vi "Extract Data.vi"(8 "Error In":errorcluster, 11 "Folder Path":path) -> (0 "Error Out":errorcluster)   [LabVIEW 2019, in "AnalysisSupport.lvlib"]
uses:
  AnalysisSupport.lvlib
  <vilib>/regexp/Match Regular Expression.xnode
  <vilib>/Analysis/NI_AALBase.lvlib
  CollectionSupport.lvlib
panel:
  out "SPL Values":dbl[](array[numeric])
  out "PTP Values":dbl[](array[numeric])
  out "Pressure Values":dbl[](array[numeric])
  out "MFR Values":dbl[](array[numeric])
  out "File Contents":string[][](array[string])
  out "File Index":i32
  out "File Match":bool
  out "Row Index":i32
  out "SPL Match":bool
  out "PTP Match":bool
  out "Pressure/SGP Match":bool
  out "MFR Match":bool
  out "All Files in Dir":path[](array[path])
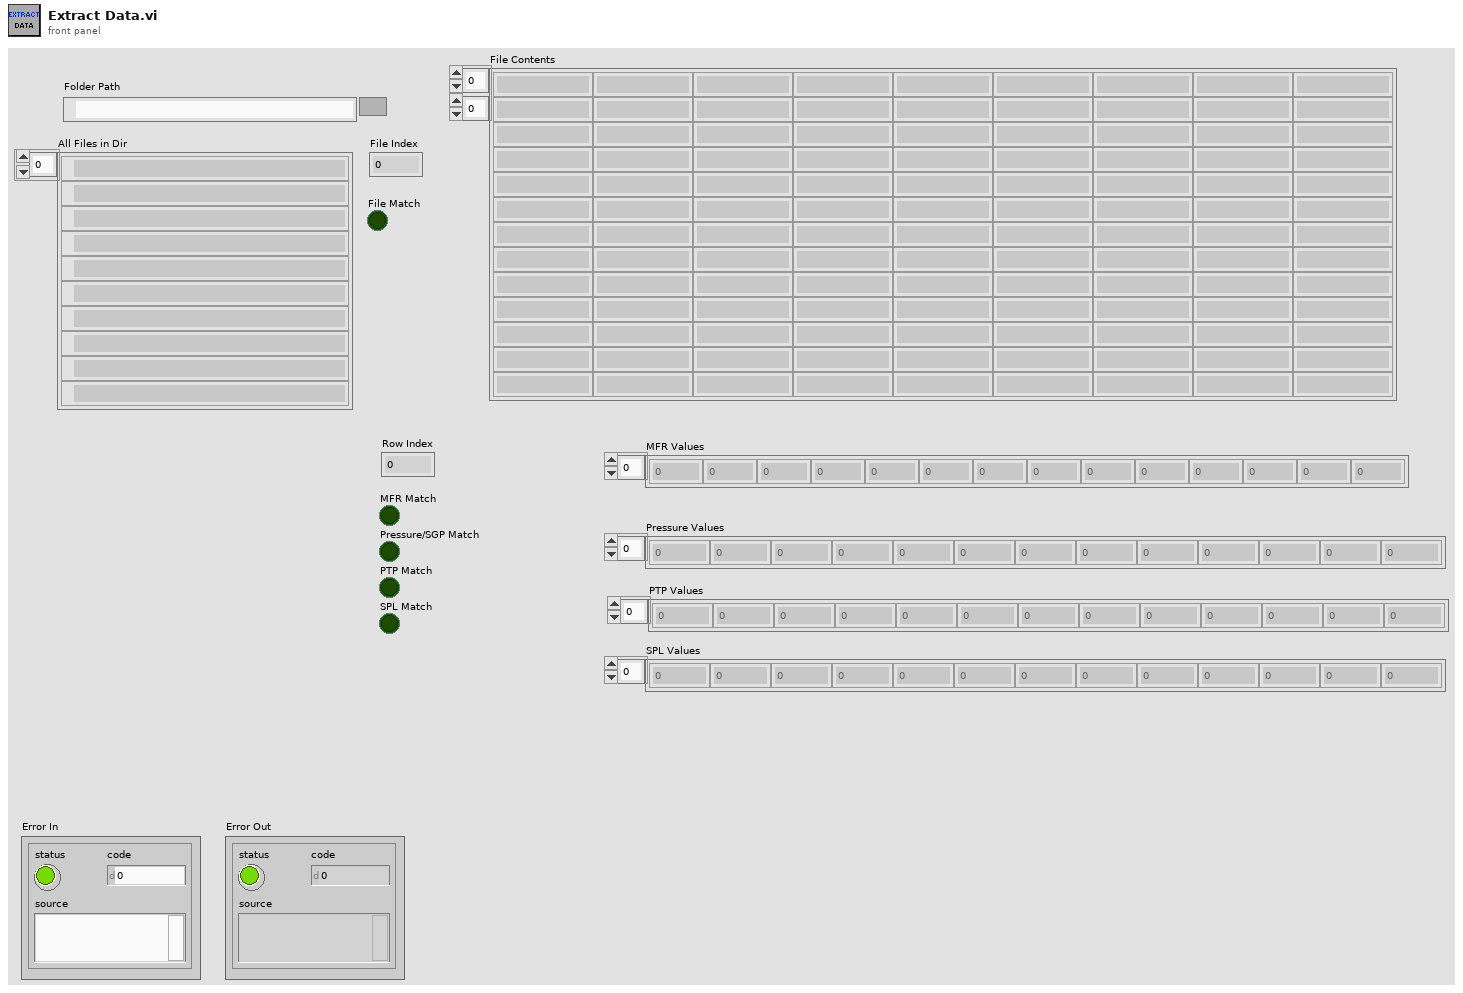
[diagram p1: front panel]
types:
  T1 = enum16{"open", "replace", "create", "open or create", "replace or create", "replace or create with confirmation"}
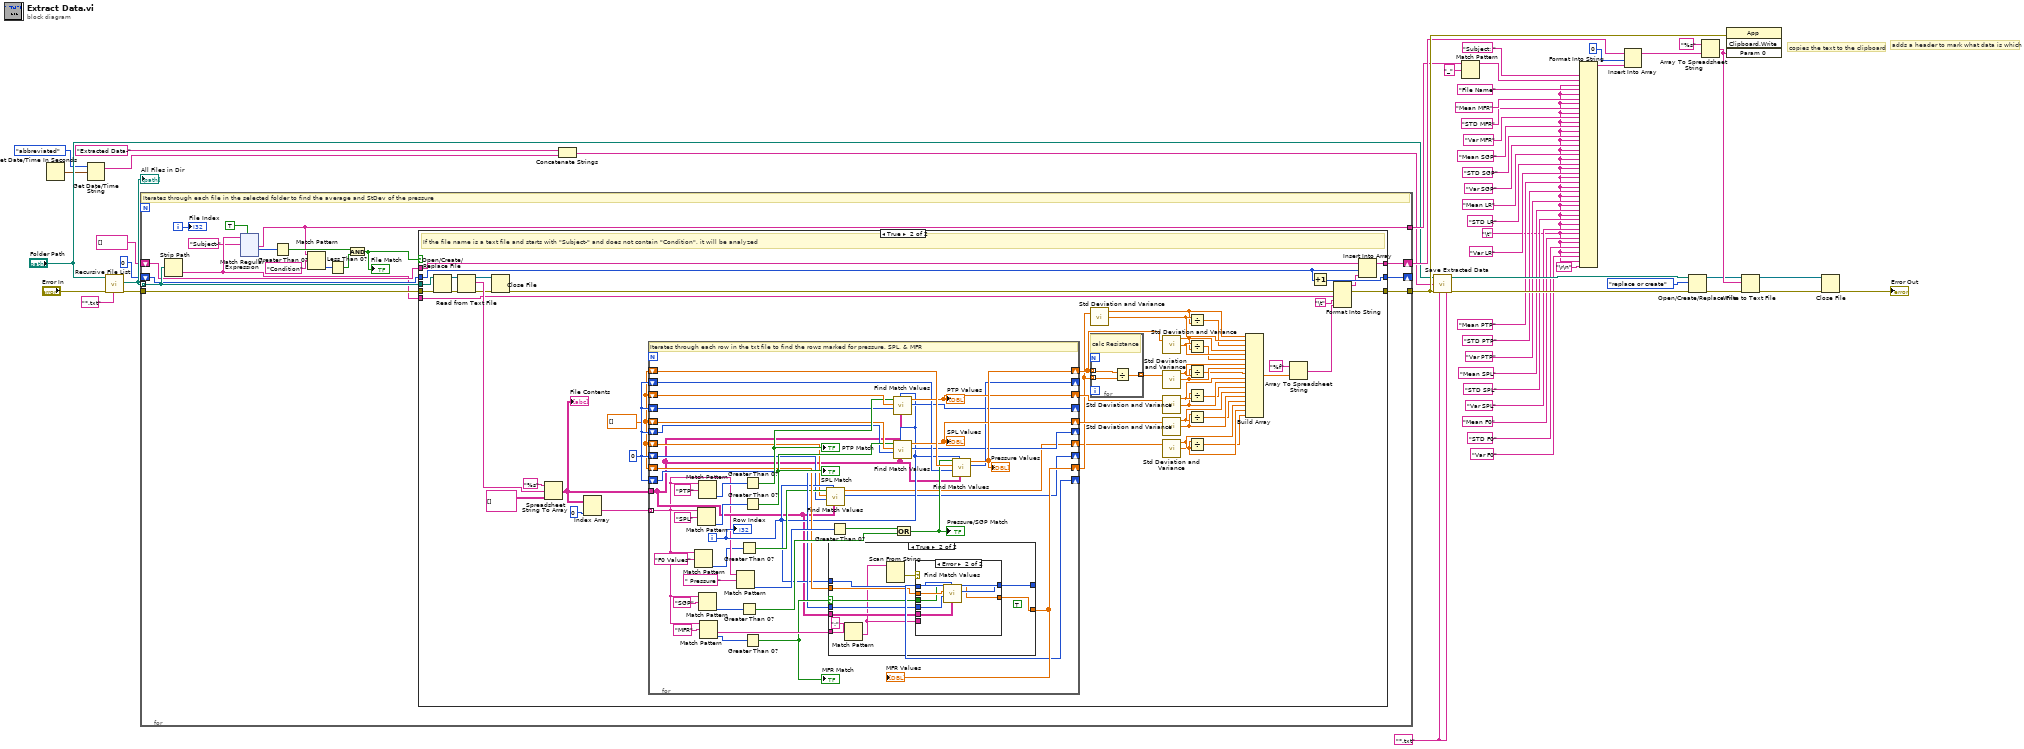
[diagram p0: block diagram]
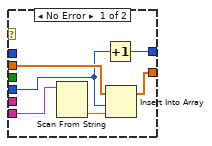
[diagram p4: hidden frame]
diagram:
  w7 = "\t"
  w42 = "*.txt" ("pattern label")
  # "adds a header to mark what data is which"
  # "copies the text to the clipboard"
  n1 = Get Date/Time In Seconds() -> (seconds since 1Jan1904=w5:timestamp)
  n2 = Get Date/Time String(date format (0)=enum16{"short", "long", "abbreviated"}."abbreviated", seconds (now)=w5) -> (date string=w3:string)  [unwired: 1 in, 1 out]
  n3 = call <vilib>:"Recursive File List.vi"("pattern"="*.txt", "error in (no error)"="Error In", "Folder Path"="Folder Path") -> ("error out"=w51:errorcluster, "All Files in Dir"=w52:path[])  [unwired: 4 in, 3 out]
  "All Files in Dir" <- w52
  n4 = for {
    tunnel: w51 -> [w70]
    tunnel: w52 -> [w69] mode=indexing
    shift-right: [w71] -> w38
    shift-left: string[] [] -> [w65]
    shift-right: [w67] -> _
    shift-left: 0 ("index") -> [w68]
    tunnel: [w66] -> w41
    tunnel: [w55] -> w35
    i -> [w54]
    # "Iterates through each file in the selected folder to find the average and StDev of the pressure"
    n5 = Strip Path(path=w69) -> (name=w58:string)  [unwired: 1 out]
    n6 = xnode "Match Regular Expression"("input string"=w58, "regular expression"="Subject-", "ignore case? (F)"=TRUE) -> ("after match"=w55:string, "offset past match"=w56:i32)  [unwired: 3 in, 3 out]
    n7 = Greater Than 0?(x=w56) -> (x > 0?=w62:bool)
    n8 = Match Pattern(string=w55, regular expression="Condition") -> (offset past match=w60:i32)  [unwired: 1 in, 3 out]
    n9 = Less Than 0?(x=w60) -> (x < 0?=w61:bool)
    n10 = And(x=w62, y=w61) -> (x .and. y?=w63:bool)
    "File Match" <- w63
    n11 = case shown="True" w63 {
      tunnel: [w188 w224] -> w71
      tunnel: w70 -> [w186 w227]
      tunnel: w65 -> [w188 w225]
      tunnel: w69 -> [_ w226]
      tunnel: w68 -> [w187 w223]
      tunnel: [w187 w222] -> w67
      tunnel: w58 -> [_ w216]
      tunnel: [w186 w213] -> w66
      frame False {
        # "If a text file doesn't match what we are looking for, nothing happens"
      }
      frame True {
        w191 = 0 ("index")
        w190 = dbl[] [] ("Array")
        # "If the file name is a text file and starts with \"Subject-\" and does not contain \"Condition\", it will be analyzed"
        n12 = Open/Create/Replace File(file path (use dialog)=w226, error in=w227) -> (refnum out=w238:refnum<file>, error out=w237:errorcluster)  [unwired: 4 in, 1 out]
        n13 = Read from Text File(file (use dialog)=w238, error in=w237) -> (refnum out=w236:refnum<file>, text=w235:string, error out=w215:errorcluster)  [unwired: 2 in, 1 out]
        n14 = Close File(refnum=w236, error in=w215) -> (error out=w214:errorcluster)  [unwired: 1 out]
        n15 = Spreadsheet String To Array(format string="%s", spreadsheet string=w235, array type (2D Dbl)=string[][] []) -> (array=w195:string[][])  [unwired: 1 in]
        "File Contents" <- w195
        n16 = Index Array(array=w195, index (col)=0 ("index (row)")) -> (element=w231:string[])  [unwired: 1 in]
        n17 = for {
          tunnel: w231 -> [w245] mode=indexing
          shift-right: [w262] -> w196
          shift-left: w190 -> [w260]
          shift-right: [w252] -> _
          shift-left: w191 -> [w253]
          tunnel: w195 -> [w247]
          shift-right: [w279] -> w197
          shift-left: w190 -> [w280]
          shift-right: [w256] -> _
          shift-left: w191 -> [w257]
          shift-right: [w269] -> w229
          shift-left: w190 -> [w273]
          shift-right: [w258] -> _
          shift-left: w191 -> [w259]
          shift-right: [w254] -> _
          shift-left: w191 -> [w255]
          shift-right: [w267] -> w228
          shift-left: w190 -> [w268]
          shift-right: [w243] -> _
          shift-left: w191 -> [w249]
          shift-right: [w242] -> w189
          shift-left: w190 -> [w248]
          i -> [w250]
          # "Iterates through each row in the txt file to find the rows marked for pressure, SPL, & MFR"
          n18 = Match Pattern(string=w245, regular expression="F0 Values") -> (offset past match=w244:i32)  [unwired: 1 in, 3 out]
          n19 = Match Pattern(string=w245, regular expression="SPL" ("element")) -> (offset past match=w266:i32)  [unwired: 1 in, 3 out]
          n20 = Match Pattern(string=w245, regular expression="PTP" ("element")) -> (offset past match=w272:i32)  [unwired: 1 in, 3 out]
          n21 = Match Pattern(string=w245, regular expression="SGP" ("element")) -> (offset past match=w282:i32)  [unwired: 1 in, 3 out]
          n22 = Match Pattern(string=w245, regular expression="MFR") -> (after substring=w263:string, offset past match=w283:i32)  [unwired: 1 in, 2 out]
          n23 = Match Pattern(string=w245, regular expression=" Pressure ") -> (offset past match=w275:i32)  [unwired: 1 in, 3 out]
          n24 = Greater Than 0?(x=w244) -> (x > 0?=w251:bool)
          n25 = Greater Than 0?(x=w282) -> (x > 0?=w278:bool)
          n26 = Greater Than 0?(x=w272) -> (x > 0?=w270:bool)
          "PTP Match" <- w270
          n27 = Greater Than 0?(x=w266) -> (x > 0?=w264:bool)
          "SPL Match" <- w264
          n28 = Greater Than 0?(x=w283) -> (x > 0?=w261:bool)
          "MFR Match" <- w261
          n29 = call "Find Match Values.vi"("Text File String"=w247, "Row Index"=w250, "New Array Index"=w249, "Blank Array"=w248, "Pattern Match?"=w251) -> ("index out"=w243:i32, "Array of Values"=w242:dbl[])  [unwired: 5 in]
          n30 = case shown="True" w261 {
            selector: w261 -> [_ w292]
            tunnel: w263 -> [_ w289]
            tunnel: w247 -> [_ w297]
            tunnel: w250 -> [_ w296]
            tunnel: w260 -> [w286 w295]
            tunnel: [w285 w294] -> w258
            tunnel: [w286 w293] -> w262
            tunnel: w259 -> [w285 w291]
            frame False {
            }
            frame True {
              (unwired) TRUE ("allow empty tokens? (F)")
              n31 = Match Pattern(string=w289, regular expression=":") -> (after substring=w288:string)  [unwired: 1 in, 3 out]
              n32 = Scan From String "Scan From String"(input string=w288) -> (error out=w290:errorcluster)  [unwired: 5 in, 2 out]
              n33 = case shown="Error" w290 {
                tunnel: w288 -> [w303 _]
                tunnel: w297 -> [_ w310]
                tunnel: w296 -> [_ w309]
                tunnel: w295 -> [w301 w308]
                tunnel: w292 -> [_ w307]
                tunnel: [w299 w306] -> w294
                tunnel: [w300 w305] -> w293
                tunnel: w291 -> [w298 w304]
                frame No Error {
                  n34 = Scan From String(input string=w303) -> (output 1=w302:dbl)  [unwired: 4 in, 3 out]
                  n35 = Increment(x=w298) -> (x+1=w299:i32)
                  n36 = Insert Into Array(array=w301, index=w298, new element=w302) -> (w300:dbl[])
                }
                frame Error {
                  n37 = call "Find Match Values.vi"("Text File String"=w310, "Row Index"=w309, "New Array Index"=w304, "Blank Array"=w308, "Pattern Match?"=w307) -> ("index out"=w306:i32, "Array of Values"=w305:dbl[])  [unwired: 5 in]
                }
              }
            }
          }
          "MFR Values" <- w262
          n38 = Greater Than 0?(x=w275) -> (x > 0?=w274:bool)
          n39 = call "Find Match Values.vi"("Text File String"=w247, "Row Index"=w250, "New Array Index"=w255, "Blank Array"=w273, "Pattern Match?"=w270) -> ("index out"=w254:i32, "Array of Values"=w269:dbl[])  [unwired: 5 in]
          "PTP Values" <- w269
          n40 = call "Find Match Values.vi"("Text File String"=w247, "Row Index"=w250, "New Array Index"=w253, "Blank Array"=w268, "Pattern Match?"=w264) -> ("index out"=w252:i32, "Array of Values"=w267:dbl[])  [unwired: 5 in]
          "SPL Values" <- w267
          n41 = Or(x=w274, y=w278) -> (x .or. y?=w277:bool)
          "Pressure/SGP Match" <- w277
          n42 = call "Find Match Values.vi"("Text File String"=w247, "Row Index"=w250, "New Array Index"=w257, "Blank Array"=w280, "Pattern Match?"=w277) -> ("index out"=w256:i32, "Array of Values"=w279:dbl[])  [unwired: 5 in]
          "Pressure Values" <- w279
          "Row Index" <- w250
        }
        n43 = call <vilib>:"Std Deviation and Variance.vi"("X"=w196) -> ("mean"=w211:dbl, "standard deviation"=w212:dbl)  [unwired: 1 in, 1 out]
        n44 = for {
          tunnel: w197 -> [w241] mode=indexing
          tunnel: w196 -> [w240] mode=indexing
          tunnel: [w239] -> w230 mode=indexing
          # "calc Resistance"
          n45 = Divide(x=w241, y=w240) -> (x/y=w239:dbl)
        }
        n46 = call <vilib>:"Std Deviation and Variance.vi"("X"=w197) -> ("mean"=w205:dbl, "standard deviation"=w206:dbl)  [unwired: 1 in, 1 out]
        n47 = call <vilib>:"Std Deviation and Variance.vi"("X"=w230) -> ("mean"=w209:dbl, "standard deviation"=w208:dbl)  [unwired: 1 in, 1 out]
        n48 = call <vilib>:"Std Deviation and Variance.vi"("X"=w229) -> ("mean"=w200:dbl, "standard deviation"=w199:dbl)  [unwired: 1 in, 1 out]
        n49 = call <vilib>:"Std Deviation and Variance.vi"("X"=w228) -> ("mean"=w202:dbl, "standard deviation"=w203:dbl)  [unwired: 1 in, 1 out]
        n50 = call <vilib>:"Std Deviation and Variance.vi"("X"=w189) -> ("mean"=w194:dbl, "standard deviation"=w193:dbl)  [unwired: 1 in, 1 out]
        n51 = Divide(x=w212, y=w211) -> (x/y=w210:dbl)
        n52 = Divide(x=w206, y=w205) -> (x/y=w204:dbl)
        n53 = Divide(x=w208, y=w209) -> (x/y=w207:dbl)
        n54 = Divide(x=w199, y=w200) -> (x/y=w198:dbl)
        n55 = Divide(x=w203, y=w202) -> (x/y=w201:dbl)
        n56 = Divide(x=w193, y=w194) -> (x/y=w192:dbl)
        n57 = Build Array(w211, w212, w210, w205, w206, w204, w209, w208, w207, w200, w199, w198, w202, w203, w201, w194, w193, w192) -> (w220:dbl[])
        n58 = Array To Spreadsheet String(array=w220, 3:"%f" ("format string")) -> (spreadsheet string=w217:string)  [unwired: 1 in]
        n59 = Increment(x=w223) -> (x+1=w222:i32)
        n60 = Format Into String(error in=w214, w216, "\t", w217) -> (resulting string=w219:string, error out=w213:errorcluster)  [unwired: 2 in]
        n61 = Insert Into Array(array=w225, index=w223, new element=w219) -> (w224:string[])
      }
    }
    "File Index" <- w54
  }
  n62 = Concatenate Strings("Extracted Data-" ("default name"), w3) -> (w2:string)
  n63 = call "Save Extracted Data"("start path"="Folder Path", "default name"=w2, "error in"=w41, "pattern (all files)"=w42, "pattern label"=w42) -> ("selected path"=w39:path, "error out"=w40:errorcluster)  [unwired: 7 in, 2 out]
  n64 = Match Pattern(string=w35, regular expression="_") -> (before substring=w32:string)  [unwired: 1 in, 3 out]
  n65 = Format Into String("Subject: " ("input 1"), w32, w7, "File Name" ("input 4"), w7, "Mean MFR" ("input 6"), w7, "STD MFR" ("input 8"), w7, "Var MFR" ("input 10"), w7, "Mean SGP" ("input 12"), w7, "STD SGP" ("input 14"), w7, "Var SGP" ("input 16"), w7, "Mean LR" ("input 18"), w7, "STD LR" ("input 20"), w7, "Var LR" ("input 22"), w7, "Mean PTP" ("input 24"), w7, "STD PTP" ("input 26"), w7, "Var PTP" ("input 28"), w7, "Mean SPL" ("input 30"), w7, "STD SPL" ("input 33"), w7, "Var SPL" ("input 35"), w7, "Mean F0" ("input 30"), w7, "STD F0" ("input 33"), w7, "Var F0" ("input 35"), w7, "\r\n") -> (resulting string=w33:string)  [unwired: 3 in, 1 out]
  n66 = Insert Into Array(array=w38, index=0, new element=w33) -> (w36:string[])
  n67 = Open/Create/Replace File(file path (use dialog)=w39, error in=w40, operation (0:open)=T1."replace or create") -> (refnum out=w47:refnum<file>, error out=w45:errorcluster)  [unwired: 3 in, 1 out]
  n68 = Array To Spreadsheet String(array=w36, 3:"%s" ("format string")) -> (spreadsheet string=w48:string)  [unwired: 1 in]
  n69 = invoke class="App" method="Clipboard.Write"(error in=w41, "Param 0"=w48) -> ()  [unwired: 2 in, 4 out]
  n70 = Write to Text File(file (use dialog)=w47, text=w48, error in=w45) -> (refnum out=w44:refnum<file>, error out=w46:errorcluster)  [unwired: 1 in, 1 out]
  n71 = Close File(refnum=w44, error in=w46) -> (error out=→"Error Out":errorcluster)  [unwired: 1 out]
